vi "DataFileCreator3.vi"(10 "ProjectName":string="QFinger", 11 "Folder path input":path=path "C:/Labview34970A stuff/Data") -> (2 "NewFileCreated":string, 3 "NewFilePath":path)   [LabVIEW 2016]
doc: "Given an input Folder path this VI creates the next data file in the format \n2017-09-17ProjectName#001\nIt only checks the latest file in the folder to decide if a sequence with today's date already exists.\nIf the file sequence has not been started, it creates one begining with #001\nIf it happens that it tries to create a file that already exists, a dialog pops up\nasking for a new name."
panel:
  out "filenames":string[](array[string])
  out "Newest file containing a #+3chars":string
  out "end of newest file name":string
  out "File time stamps sorted by time":timestamp[](array[timestamp])
  out "Files in Folder sorted by time":path[](array[path])
  out "FileTypeExists?":bool
  out "date string":string
  out "YearNow":string
  out "DayNow":string
  out "MonthNow":string
  out "DayParsed":string
  out "MonthParsed":string
  out "YearParsed":string
  out "newest existing file":string
  # "Given an input Folder path this VI creates the next data file in the format \n2017-09-17ProjectName#001\nIt only checks the latest file in the folder to decide if \na sequence with today's date already exists.\nIf the file sequence has not been started, it creates one begining with #001\nIf it happens that it tries to create a file that already exists, a dialog pops up\nasking for a new name.\n2017 11 07- now this finds the newest file containing a # so it doesn't get confused if\nthere is a log file that is newer than the latest data file"
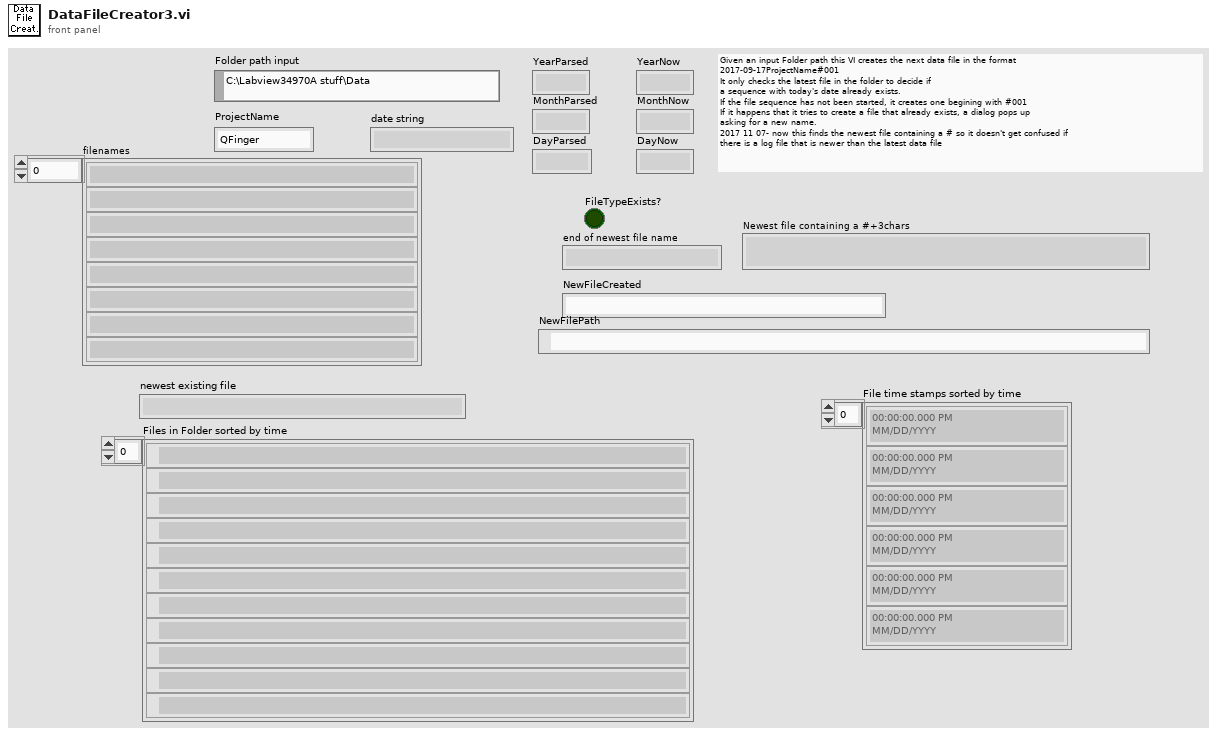
[diagram p1: front panel]
types:
  T1 = enum16{"open", "replace", "create", "open or create", "replace or create", "replace or create with confirmation"}
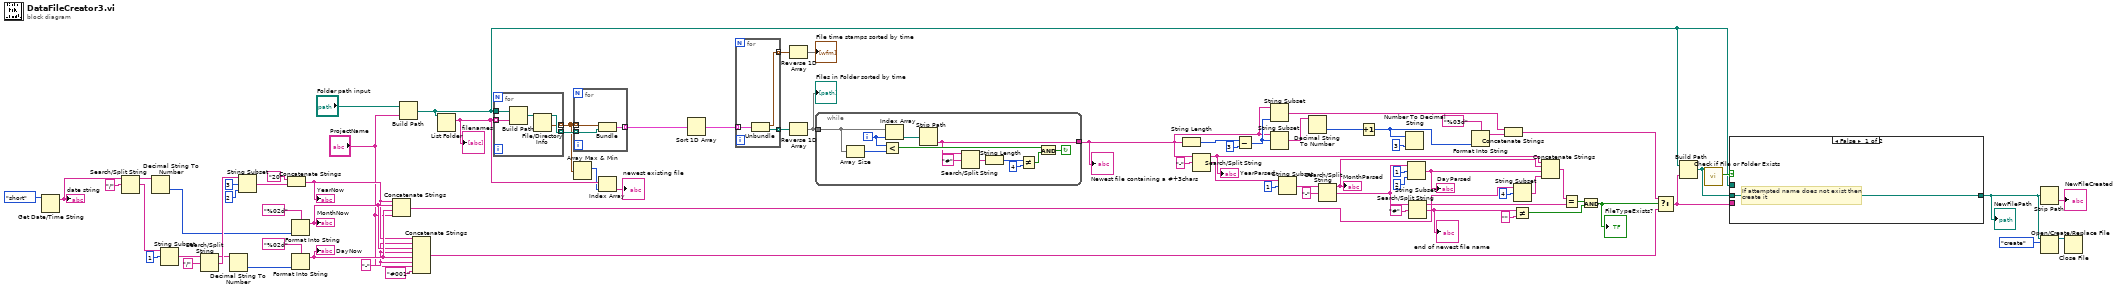
[diagram p0: block diagram]
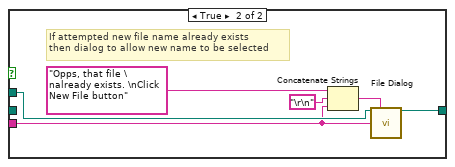
[diagram p2: hidden frame]
diagram:
  w45 = "-" ("string")
  n1 = Get Date/Time String(date format (0)=enum16{"short", "long", "abbreviated"}."short") -> (date string=w61:string)  [unwired: 2 in, 1 out]
  "date string" <- w61
  n2 = Search/Split String(string=w61, search string/char (-)="/") -> (substring before match=w55:string, match + rest of string=w69:string)  [unwired: 1 in, 1 out]
  n3 = Decimal String To Number(string=w55) -> (number=w54:i32)  [unwired: 2 in, 1 out]
  n4 = String Subset(string=w69, offset (0)=1) -> (substring=w68:string)  [unwired: 1 in]
  n5 = Search/Split String(string=w68, search string/char (-)="/") -> (substring before match=w51:string, match + rest of string=w66:string)  [unwired: 1 in, 1 out]
  n6 = Decimal String To Number(string=w51) -> (number=w52:i32)  [unwired: 2 in, 1 out]
  n7 = String Subset(string=w66, offset (0)=3, length (rest)=2 ("y")) -> (substring=w63:string)
  n8 = Concatenate Strings("20" ("string"), w63) -> (w46:string)
  "YearNow" <- w46
  n9 = Format Into String(format string="%02d", w54) -> (resulting string=w47:string)  [unwired: 2 in, 1 out]
  "MonthNow" <- w47
  n10 = Format Into String(format string="%02d", w52) -> (resulting string=w48:string)  [unwired: 2 in, 1 out]
  "DayNow" <- w48
  n11 = Concatenate Strings(w46, w47, w48, "ProjectName") -> (w57:string)
  n12 = Build Path(base path="Folder path input", name or relative path="ProjectName") -> (appended path=w2:path)
  n13 = Concatenate Strings(w46, w45, w47, w45, w48, w45, "ProjectName", "#001" ("string")) -> (w42:string)
  n14 = List Folder(path=w2) -> (filenames=w8:string[])  [unwired: 3 in, 3 out]
  "filenames" <- w8
  n15 = for {
    tunnel: w8 -> [w84] mode=indexing
    tunnel: [w82] -> w20 mode=indexing
    tunnel: [w81] -> w19 mode=indexing
    tunnel: w2 -> [w80]
    n16 = Build Path(base path=w80, name or relative path=w84) -> (appended path=w83:path)
    n17 = File/Directory Info(path=w83) -> (path out=w82:path, last mod=w81:timestamp)  [unwired: 1 in, 5 out]
  }
  n18 = for {
    tunnel: w19 -> [w87] mode=indexing
    tunnel: w20 -> [w86] mode=indexing
    tunnel: [w85] -> w24 mode=indexing
    n19 = Bundle("last mod"=w87, "path out"=w86) -> (w85:cluster{"last mod":timestamp, "path out":path})  [unwired: 1 in]
  }
  n20 = Array Max & Min(array=w19) -> (max index (indices)=w7:i32)  [unwired: 3 out]
  n21 = Index Array(array=w8, index=w7) -> (element=→"newest existing file":string)
  n22 = Sort 1D Array(array=w24) -> (sorted array=w23:cluster{"last mod":timestamp, "path out":path}[])
  n23 = for {
    tunnel: w23 -> [w90] mode=indexing
    tunnel: [w89] -> w6 mode=indexing
    tunnel: [w88] -> w22 mode=indexing
    n24 = Unbundle(w90) -> ("last mod"=w88:timestamp, "path out"=w89:path)
  }
  n25 = Reverse 1D Array(array=w22) -> (reversed array=→"File time stamps sorted by time":timestamp[])
  n26 = Reverse 1D Array(array=w6) -> (reversed array=w5:path[])
  "Files in Folder sorted by time" <- w5
  n27 = while {
    tunnel: w5 -> [w100]
    tunnel: [w95] -> w4
    i -> [w98]
    stop <- w101 continue-if-true
    n28 = Array Size(array=w100) -> (size(s)=w99:i32)
    n29 = Less?(x=w98, y=w99) -> (x < y?=w97:bool)
    n30 = Index Array(array=w100, index=w98) -> (element=w96:path)
    n31 = Strip Path(path=w96) -> (name=w95:string)  [unwired: 1 out]
    n32 = Search/Split String(string=w95, search string/char (-)="#") -> (match + rest of string=w94:string)  [unwired: 1 in, 2 out]
    n33 = String Length(string=w94) -> (length=w93:i32)
    n34 = Not Equal?(x=w93, y=4) -> (x != y?=w91:bool)
    n35 = And(x=w97, y=w91) -> (x .and. y?=w101:bool)
  }
  "Newest file containing a #+3chars" <- w4
  n36 = String Length(string=w4) -> (length=w41:i32)
  n37 = Search/Split String(string=w4, search string/char (-)="-") -> (substring before match=w49:string, match + rest of string=w76:string)  [unwired: 1 in, 1 out]
  "YearParsed" <- w49
  n38 = Subtract(x=w41, y=3) -> (x-y=w39:i32)
  n39 = String Subset(string=w4, length (rest)=w39) -> (substring=w33:string)  [unwired: 1 in]
  n40 = String Subset(string=w4, offset (0)=w39) -> (substring=w38:string)  [unwired: 1 in]
  n41 = String Subset(string=w76, offset (0)=1) -> (substring=w75:string)  [unwired: 1 in]
  n42 = Decimal String To Number(string=w38) -> (number=w37:i32)  [unwired: 2 in, 1 out]
  n43 = Search/Split String(string=w75, search string/char (-)="-") -> (substring before match=w60:string, match + rest of string=w16:string)  [unwired: 1 in, 1 out]
  "MonthParsed" <- w60
  n44 = Increment(x=w37) -> (x+1=w35:i32)
  n45 = Number To Decimal String(number=w35, width (-)=i16 3) -> ()  [unwired: 1 out]
  n46 = String Subset(string=w16, offset (0)=1, length (rest)=2 ("y")) -> (substring=w59:string)
  "DayParsed" <- w59
  n47 = Search/Split String(string=w16, search string/char (-)="#") -> (substring before match=w15:string, match + rest of string=w13:string)  [unwired: 1 in, 1 out]
  "end of newest file name" <- w13
  n48 = Format Into String(format string="%03d", w35) -> (resulting string=w32:string)  [unwired: 2 in, 1 out]
  n49 = Concatenate Strings(w33, w32) -> (w43:string)
  n50 = String Subset(string=w15, offset (0)=4) -> (substring=w14:string)  [unwired: 1 in]
  n51 = Not Equal?(x=w13, y="") -> (x != y?=w11:bool)
  n52 = Concatenate Strings(w49, w60, w59, w14) -> (w58:string)
  n53 = Equal?(x=w58, y=w57) -> (x = y?=w10:bool)
  n54 = And(x=w10, y=w11) -> (x .and. y?=w9:bool)
  "FileTypeExists?" <- w9
  n55 = Select(t=w43, s=w9, f=w42) -> (s? t:f=w27:string)
  n56 = Build Path(base path=w2, name or relative path=w27) -> (appended path=w31:path)
  n57 = call <vilib>:"Check if File or Folder Exists.vi"("path"=w31) -> ("file or folder exists?"=w30:bool)  [unwired: 8 in, 2 out]
  n58 = case shown="False" w30 {
    tunnel: w31 -> [w103 _]
    tunnel: w2 -> [_ w109]
    tunnel: [w103 w108] -> w25
    tunnel: w27 -> [_ w104]
    frame False {
      # "If attempted name does not exist then \ncreate it"
    }
    frame True {
      # "If attempted new file name already exists\nthen dialog to allow new name to be selected"
      n59 = Concatenate Strings("Opps, that file \nalready exists. \nClick New File button" ("prompt"), "\r\n", w104) -> (w105:string)
      n60 = call "File Dialog"("start path"=w109, "prompt"=w105, "default name"=w104) -> ("selected path"=w108:path)  [unwired: 9 in, 3 out]
    }
  }
  "NewFilePath" <- w25
  n61 = Strip Path(path=w25) -> (name=→"NewFileCreated":string)  [unwired: 1 out]
  n62 = Open/Create/Replace File(file path (use dialog)=w25, operation (0:open)=T1."create") -> (refnum out=w28:refnum<file>)  [unwired: 4 in, 2 out]
  n63 = Close File(refnum=w28) -> ()  [unwired: 1 in, 2 out]
